vi "Assign Overall Pass Fail.vi"(8 "error in (no error)":errorcluster, 9 "Channel":i32, 10 "Record Array in":T1[](array[typedef])=[{"Reference Value"=2.2867484949728984e-05, "Measured Value"=4.946674027466586, "Error"=4.946651159981635, "Pass/Fail"=FALSE, "Setpoint"=-1.4252255170268712e-05, "Cycle Number"=1, "Direction"=enum."Descending", "Test Status"=enum."Overall Pass"}, {"Reference Value"=2.2867484949728984e-05, "Measured Value"=4.946674027466586, "Error"=4.946651159981635, "Pass/Fail"=FALSE, "Setpoint"=-1.4252255170268712e-05, "Cycle Number"=1, "Direction"=enum."Descending", "Test Status"=enum."Overall Pass"}], 11 "New Processed Calibration Point in":T1) -> (0 "error out":errorcluster, 3 "Record Array out":T1[](array[typedef]))   [LabVIEW 2026, in "Processing_Engine.lvlib"]
uses:
  Processing_Engine.lvlib
  controls/Messaging Payloads/Processed Calibration Point.ctl
  controls/UI/Direction.ctl
  Test Status.ctl
  Analysis/Analysis.lvlib
  Settings/Settings.lvlib
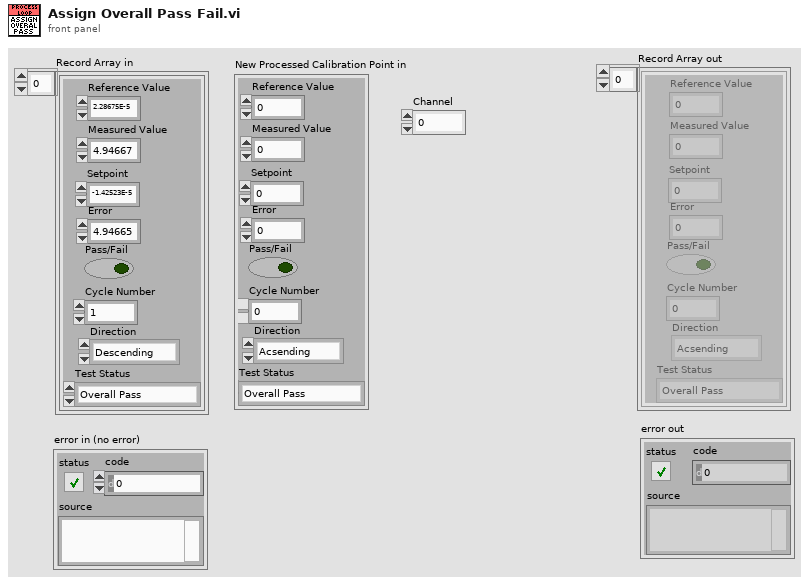
[diagram p1: front panel]
types:
  T1 = typedef "Processed Calibration Point.ctl" = cluster{"Reference Value":dbl, "Measured Value":dbl, "Error":dbl, "Pass/Fail":bool, "Setpoint":dbl, "Cycle Number":i32, "Direction":T2, "Test Status":T3}
  T2 = typedef "Settings.lvlib/Direction.ctl" = enum16{"Acsending", "Descending"}
  T3 = typedef "Analysis.lvlib/Test Status.ctl" = enum16{"Overall Pass", "Overall Fail", "Test Running"}
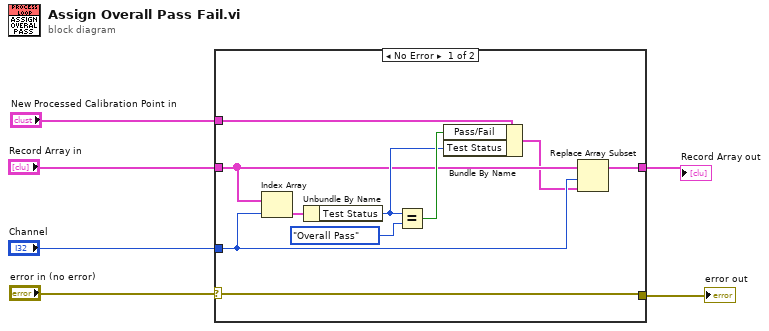
[diagram p0: block diagram]
diagram:
  n1 = case shown="No Error" "error in (no error)" {
    selector: "error in (no error)" -> [w16 w18]
    tunnel: [w16 w18] -> w5
    tunnel: "Record Array in" -> [w10 w17]
    tunnel: "Channel" -> [w9 _]
    tunnel: "New Processed Calibration Point in" -> [w14 _]
    tunnel: [w7 w17] -> w1
    frame No Error {
      n2 = Index Array(array=w10, index=w9) -> (element=w15:T1)
      n3 = Unbundle By Name(w15) -> ("Test Status"=w11:T3)
      n4 = Equal?(x=w11, y=Test_Status."Overall Pass") -> (x = y?=w12:bool)
      n5 = Bundle By Name(cluster=w14, "Pass/Fail"=w12, "Test Status"=w11) -> (w8:T1)
      n6 = Replace Array Subset(array=w10, new element=w8, index=w9) -> (w7:T1[])
    }
    frame Error {
    }
  }
  "error out" <- w5
  "Record Array out" <- w1
